vi "GetPktLoss.vi"(8 "error in (no error)":errorcluster, 11 "NetworkPlugin in":refnum<class "NetworkPlugin.lvclass">) -> (0 "error out":errorcluster, 3 "NetworkPlugin out":refnum<class "NetworkPlugin.lvclass">)   [LabVIEW 2017, in "NetworkImpairmentPlugins.lvlib" / "NetworkPlugin.lvclass"]
uses:
  NetworkPlugin.lvclass
  C:/dev/Work/PARTF/Modules/NetworkImpairmentPlugins/NetworkImpairmentPluginBase_class/NetworkImpairmentPluginBase.lvclass
  NetworkImpairmentPluginBase_class/Accessors/Read TimeArray.vi
  NetworkImpairmentPluginBase_class/Accessors/Read NetImpParams.vi
  NetworkImpairmentPluginBase_class/Accessors/Set PktLoss.vi
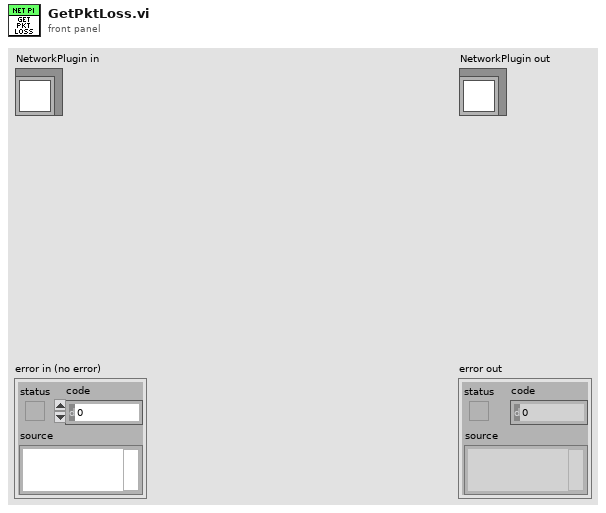
[diagram p1: front panel]
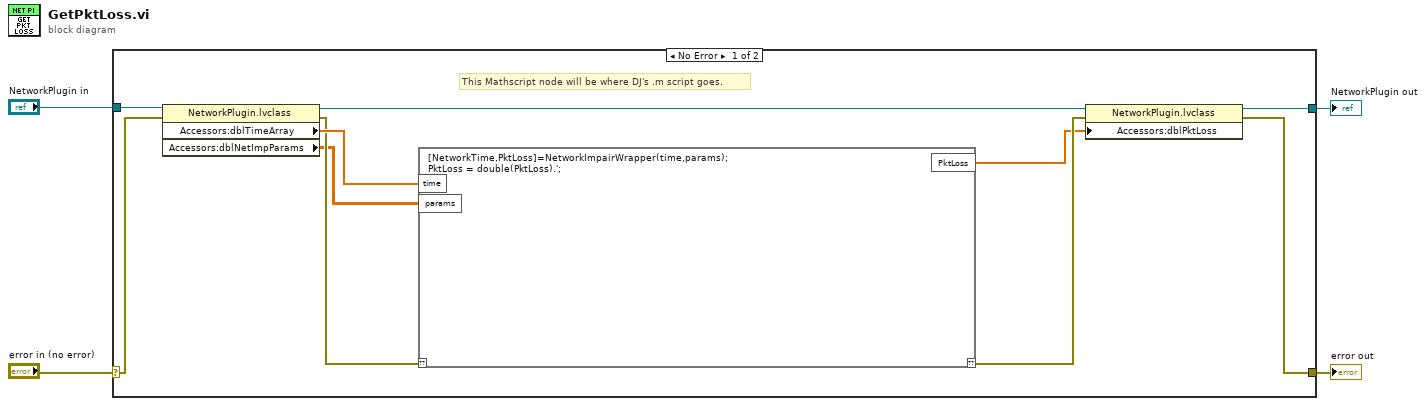
[diagram p0: block diagram]
diagram:
  n1 = case shown="No Error" "error in (no error)" {
    selector: "error in (no error)" -> [w11 w16]
    tunnel: [w10 w16] -> w1
    tunnel: [w14 w15] -> w2
    tunnel: "NetworkPlugin in" -> [w7 w15]
    frame No Error {
      # "This Mathscript node will be where DJ's .m script goes."
      n2 = property class="NetworkPlugin.lvclass"(reference=w7, error in=w11) -> (reference out=w13:refnum<class "NetworkPlugin.lvclass">, error out=w9:errorcluster, "Accessors:dblTimeArray"=w12:dbl[], "Accessors:dblNetImpParams"=w6:dbl[][])
      n3 = script code="[NetworkTime,PktLoss]=NetworkImpairWrapper(time,params);\nPktLoss = double(PktLoss).';"("??"=w9, "time"=w12, "params"=w6) -> ("??"=w8:errorcluster, "PktLoss"=w5:dbl[])
      n4 = property class="NetworkPlugin.lvclass"(reference=w13, error in=w8, "Accessors:dblPktLoss"=w5) -> (reference out=w14:refnum<class "NetworkPlugin.lvclass">, error out=w10:errorcluster)
    }
    frame Error {
    }
  }
  "error out" <- w1
  "NetworkPlugin out" <- w2
